vi "Control Type.vi"(11 "Valve in":refnum<class "DiscreteRangeControl.lvclass">) -> (2 "Valve Type":string)   [LabVIEW 2020, in "VolatusControl.lvlib" / "DiscreteRangeControl.lvclass"]
uses:
  DiscreteRangeControl.lvclass
  DiscreteRangeControl.lvclass/DiscreteRangeControl.ctl
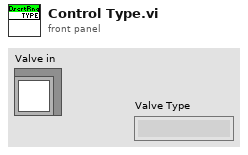
[diagram p1: front panel]
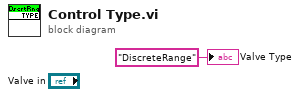
[diagram p0: block diagram]
diagram:
  "Valve Type" <- "DiscreteRange" ("Valve Type")
